vi "Launch As Nested.vi"(8 "error in (no error)":errorcluster, 11 "Parent in":refnum<class "Module.lvclass">) -> (0 "error out":errorcluster, 2 "TimerAPI":refnum<class "TimerAPI.lvclass">, 3 "Parent out":refnum<class "Module.lvclass">)   [LabVIEW 2020, in "Volatus.lvlib" / "Timing Module.lvclass"]
uses:
  Timing Module.lvclass
  Timing Module.lvclass/Timing Module.ctl
  Module/Module.lvclass
  VolatusConfig/VolatusConfigElement/VolatusConfigElement.lvclass
  C:/dev/lv20CE/relink/lv-volatus/Volatus/Module/Module.lvclass
  C:/dev/lv20CE/relink/lv-volatus/Volatus/Timing Module/Timing Module.lvclass
  TimerAPI/TimerAPI.lvclass
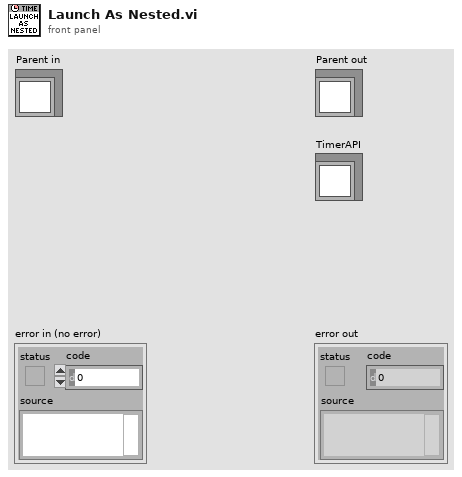
[diagram p1: front panel]
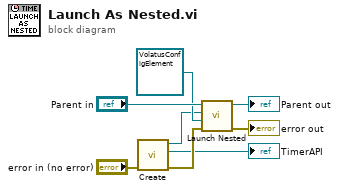
[diagram p0: block diagram]
diagram:
  n1 = call "Create.vi"("error in (no error)"="error in (no error)") -> ("error out"=w8:errorcluster, "TimerAPI"=→"TimerAPI":refnum<class "TimerAPI.lvclass">, "Timing Module out"=w4:refnum<class "Timing Module.lvclass">)  [unwired: 8 in]
  n2 = call "Launch Nested.vi"("error in (no error)"=w8, "Config Element"=refnum<class "VolatusConfigElement.lvclass"> refnum, "Nested Module"=w4, "Parent in"="Parent in") -> ("error out"=→"error out":errorcluster, "Parent out"=→"Parent out":refnum<class "Module.lvclass">)  [unwired: 5 in, 1 out]
